vi "Add VIs To Tree_No Parents.vi"(8 "error in":errorcluster, 11 "state in":T1) -> (0 "error out":errorcluster, 3 "state out":T1)   [LabVIEW 2010, in "NI_SE_Config Front Panel Layout.lvlib"]
uses:
  NI_SE_Config Front Panel Layout.lvlib
  State.ctl
  VI Info.ctl
  VI Panel Layout/VI Panel Layout.lvclass
  VI Panel Layout/VI Panel Layout.lvclass/VI Panel Layout.ctl
  VI Panel Layout/Get Subpanel VIs.vi
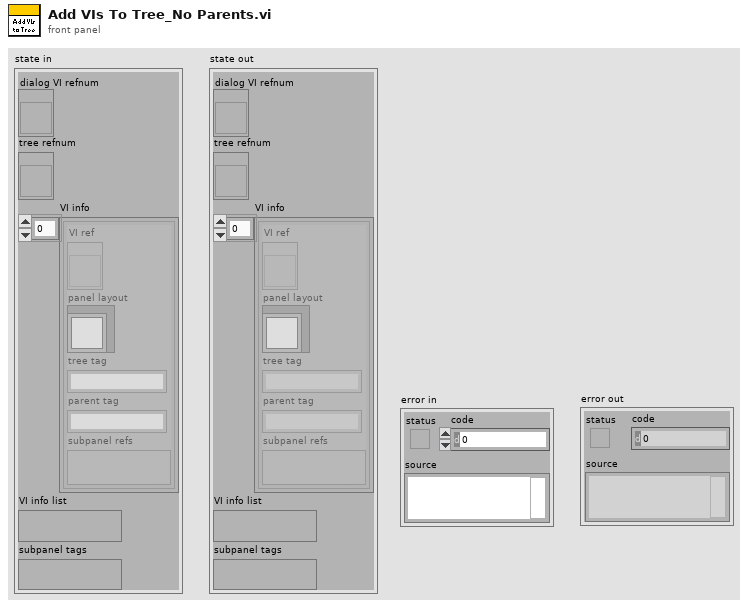
[diagram p1: front panel]
types:
  T1 = typedef "NI_SE_Config Front Panel Layout.lvlib/State.ctl" = cluster{"dialog VI refnum":refnum<vi>, "tree refnum":refnum<vi>, "VI info":T2[], "VI info list":variant, "subpanel tags":variant}
  T2 = typedef "NI_SE_Config Front Panel Layout.lvlib/VI Info.ctl" = cluster{"VI ref":refnum<vi>, "panel layout":refnum<class "VI Panel Layout.lvclass">, "tree tag":string, "parent tag":string, "subpanel refs":variant}
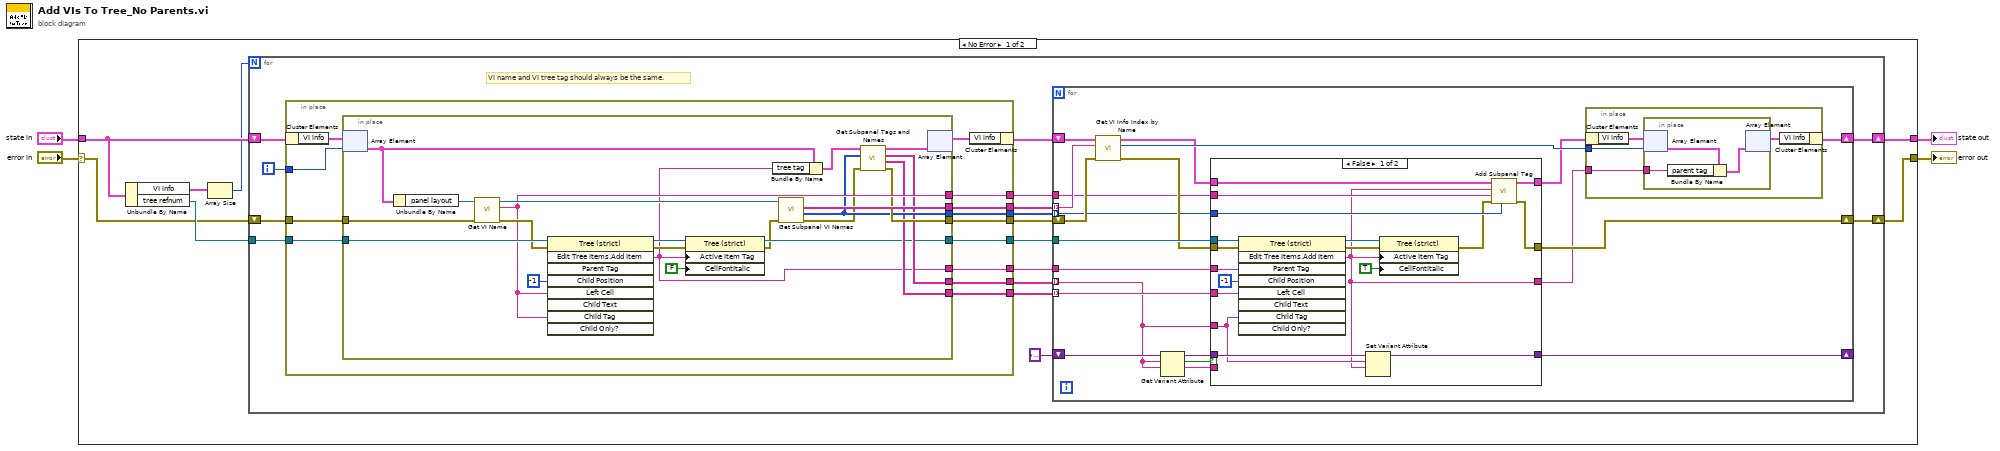
[diagram p0: block diagram]
diagram:
  n1 = case shown="No Error" "error in" {
    selector: "error in" -> [w7 w113]
    tunnel: "state in" -> [w10 w114]
    tunnel: [w6 w114] -> w2
    tunnel: [w5 w113] -> w1
    frame No Error {
      n2 = Unbundle By Name(w10) -> ("VI info"=w11:T2[], "tree refnum"=w8:refnum<vi>)
      n3 = Array Size(array=w11) -> (size(s)=w9:i32)
      n4 = for {
        N: w9 -> [_]
        shift-right: [w18] -> w5
        shift-left: w7 -> [w26]
        tunnel: w8 -> [w27]
        shift-right: [w21] -> w6
        shift-left: w10 -> [w25]
        i -> [w24]
        # "VI name and VI tree tag should always be the same."
        n5 = in-place {
          in-place-border: w27 -> [w90]
          in-place-border: w26 -> [w89]
          in-place-border: [w88] -> w20
          in-place-border: w24 -> [w82]
          in-place-border: [w85] -> w19
          in-place-border: [w84] -> w23
          in-place-border: [w83] -> w17
          in-place-border: [w81] -> w16
          in-place-border: [w80] -> w14
          in-place-border: [w79] -> w13
          in-place-border: [w78] -> w12
          n6 = in-place-cluster #1(w25) -> ("VI info"=w87:T2[])
          n7 = in-place {
            in-place-border: w90 -> [w111]
            in-place-border: w89 -> [w110]
            in-place-border: [w101] -> w88
            in-place-border: [w92] -> w85
            in-place-border: [w107] -> w84
            in-place-border: [w100] -> w83
            in-place-border: [w95] -> w81
            in-place-border: [w104] -> w80
            in-place-border: [w99] -> w79
            in-place-border: [w98] -> w78
            n8 = in-place-array #2(w87, w82) -> (w108:T2)
            n9 = Unbundle By Name(w108) -> ("panel layout"=w112:refnum<class "VI Panel Layout.lvclass">)
            n10 = call "Get VI Name.vi"("error in (no error)"=w110, "VI Panel Layout in"=w112) -> ("error out"=w106:errorcluster, "VI name"=w104:string, "VI Panel Layout out"=w109:refnum<class "VI Panel Layout.lvclass">)  [unwired: 7 in]
            n11 = invoke class="Tree (strict)" method="Edit Tree Items.Add Item"(reference=w111, error in=w106, "Child Position"=-1, "Left Cell"=w104, "Child Tag"=w104) -> (reference out=w96:refnum<vi>, error out=w94:errorcluster, "Edit Tree Items:Add Item"=w92:string)  [unwired: 4 in, 6 out]
            n12 = property class="Tree (strict)"(reference=w96, error in=w94, "Active Item Tag"=w92, "CellFontItalic"=FALSE ("Active Cell:Cell Font:Italic")) -> (reference out=w95:refnum<vi>, error out=w93:errorcluster)
            n13 = Bundle By Name(cluster=w108, "tree tag"=w92) -> (w103:T2)
            n14 = call "Get Subpanel VI Names.vi"("error in (no error)"=w93, "VI Panel Layout in"=w109) -> ("error out"=w97:errorcluster, "subpanel object UIDs"=w100:i32[], "VI names"=w107:string[])  [unwired: 5 in, 2 out]
            n15 = call "Get Subpanel Tags and Names.vi"("error in"=w97, "subpanel UIDs"=w100, "VI info in"=w103) -> ("error out"=w101:errorcluster, "subpanel names"=w98:string[], "subpanel tags"=w99:string[], "VI info out"=w102:T2)  [unwired: 5 in]
            n16 = in-place-array #2(w102) -> (w86:T2[])  [unwired: 1 out]
          }
          n17 = in-place-cluster #1("VI info"=w86) -> (w22:T1)
        }
        n18 = for {
          tunnel: w23 -> [w47] mode=indexing
          shift-right: [w46] -> w21
          shift-left: w22 -> [w48]
          shift-right: [w41] -> w18
          shift-left: w20 -> [w43]
          tunnel: w19 -> [w40]
          tunnel: w17 -> [w31] mode=indexing
          tunnel: w16 -> [w44]
          shift-right: [w34] -> _
          shift-left: variant -> [w38]
          tunnel: w14 -> [w30]
          tunnel: w13 -> [w28] mode=indexing
          tunnel: w12 -> [w29] mode=indexing
          n19 = call "Get VI Info Index by Name.vi"("error in"=w43, "VI name"=w47, "state in"=w48) -> ("error out"=w42:errorcluster, "VI info index"=w45:i32, "state out"=w33:T1)  [unwired: 5 in, 1 out]
          n20 = Get Variant Attribute(Variant=w38, name=w28, default value (empty Variant)=w28) -> (duplicate Variant=w37:variant, found=w36:bool, value=w35:string)  [unwired: 1 in, 1 out]
          n21 = case shown="False" w36 {
            tunnel: w44 -> [w66 _]
            tunnel: w42 -> [w65 w70]
            tunnel: [w58 w70] -> w41
            tunnel: w40 -> [w64 _]
            tunnel: w28 -> [w62 _]
            tunnel: [w49 w69] -> w39
            tunnel: w37 -> [w63 w68]
            tunnel: w35 -> [_ w69]
            tunnel: [w61 w68] -> w34
            tunnel: w33 -> [w60 w67]
            tunnel: [w59 w67] -> w32
            tunnel: w31 -> [w57 _]
            tunnel: w30 -> [w56 _]
            tunnel: w29 -> [w54 _]
            frame False {
              n22 = invoke class="Tree (strict)" method="Edit Tree Items.Add Item"(reference=w66, error in=w65, "Parent Tag"=w64, "Child Position"=-1, "Left Cell"=w54, "Child Tag"=w62) -> (reference out=w52:refnum<vi>, error out=w51:errorcluster, "Edit Tree Items:Add Item"=w49:string)  [unwired: 3 in, 6 out]
              n23 = Set Variant Attribute(Variant=w63, name=w62, value=w49) -> (Variant out=w61:variant)  [unwired: 1 in, 2 out]
              n24 = property class="Tree (strict)"(reference=w52, error in=w51, "Active Item Tag"=w49, "CellFontItalic"=TRUE ("Active Cell:Cell Font:Italic")) -> (error out=w50:errorcluster)  [unwired: 1 out]
              n25 = call "Add Subpanel Tag.vi"("subpanel UID"=w57, "error in"=w50, "owning VI name"=w56, "subpanel tag"=w49, "state in"=w60) -> ("error out"=w58:errorcluster, "state out"=w59:T1)  [unwired: 5 in]
            }
            frame True {
            }
          }
          n26 = in-place {
            in-place-border: w45 -> [w73]
            in-place-border: w39 -> [w71]
            n27 = in-place-cluster #3(w32) -> ("VI info"=w74:T2[])
            n28 = in-place {
              in-place-border: w71 -> [w76]
              n29 = in-place-array #4(w74, w73) -> (w77:T2)
              n30 = Bundle By Name(cluster=w77, "parent tag"=w76) -> (w75:T2)
              n31 = in-place-array #4(w75) -> (w72:T2[])  [unwired: 1 out]
            }
            n32 = in-place-cluster #3("VI info"=w72) -> (w46:T1)
          }
        }
      }
    }
    frame Error {
    }
  }
  "state out" <- w2
  "error out" <- w1
